vi "PatchExtractor.vi"(8 "error in":errorcluster caption="entrée d'erreur", 11 "PatchExtractor":T1={"patch_size"={"patch_height"=0, "patch_width"=0}, "max_patches"="None", "random_state"=-1} {"random_state" min=-1}) -> (0 "error out":errorcluster caption="sortie d'erreur", 3 "PatchExtractor.lvclass":refnum<class "PatchExtractor.lvclass">)   [LabVIEW 2020]
uses:
  PatchExtractor.lvclass
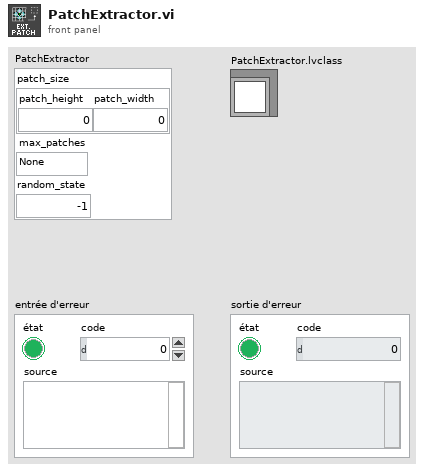
[diagram p1: front panel]
types:
  T1 = cluster{"patch_size":cluster{"patch_height":i32, "patch_width":i32}, "max_patches":string, "random_state":i32}
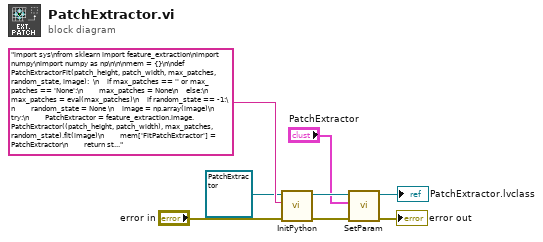
[diagram p0: block diagram]
diagram:
  n1 = call-dynamic "InitPython.vi"("error in (no error)"="error in", "Python Instruction"="import sys\nfrom sklearn import feature_extraction\nimport numpy\nimport numpy as np\n\n\nmem = {}\n\ndef PatchExtractorFit(patch_height, patch_width, max_patches, random_state, image):  \n    if max_patches == '' or max_patches == 'None':\n        max_patches = None\n    else:\n        max_patches = eval(max_patches)\n    if random_state == -1:\n        random_state = None \n    image = np.array(image)\n    try:\n        PatchExtractor = feature_extraction.image.PatchExtractor((patch_height, patch_width), max_patches, random_state).fit(image)\n        mem['FitPatchExtractor'] = PatchExtractor\n        return str('OK')\n    except:\n        erreur = sys.exc_info()\n        typerr = u\"%s\" % (erreur[0])\n        typerr = typerr[typerr.find(\"'\")+1:typerr.rfind(\"'\")]\n        msgerr = u\"%s\" % (erreur[1])\n        message = str('/!\\\\ {0} : {1}'. format(typerr,msgerr))\n        return message\n    \ndef PatchExtractorTransform(patch_height, patch_width, max_patches, random_state, image):  \n    if max_patches == '' or max_patches == 'None':\n        max_patches = None\n    else:\n        max_patches = eval(max_patches)\n    if random_state == -1:\n        random_state = None \n    image = np.array(image)\n    try:\n        Patches2D = mem['FitPatchExtractor'].transform(image)\n        Patches2Dlist = Patches2D.tolist()\n        return str(Patches2Dlist)\n    except:\n        erreur = sys.exc_info()\n        typerr = u\"%s\" % (erreur[0])\n        typerr = typerr[typerr.find(\"'\")+1:typerr.rfind(\"'\")]\n        msgerr = u\"%s\" % (erreur[1])\n        message = str('/!\\\\ {0} : {1}'. format(typerr,msgerr))\n        return message", "Scikit-learn en entrée"=refnum<class "PatchExtractor.lvclass"> refnum ("PatchExtractor.lvclass")) -> ("error out"=w5:errorcluster, "Scikit-learn en sortie"=w4:refnum<class "PatchExtractor.lvclass">)  [unwired: 7 in]
  n2 = call-dynamic "SetParam.vi"("error in (no error)"=w5, "PatchExtractor"="PatchExtractor", "PatchExtractor.lvclass"=w4) -> ("error out"=→"error out":errorcluster, "PatchExtractor.lvclass"=→"PatchExtractor.lvclass":refnum<class "PatchExtractor.lvclass">)  [unwired: 7 in]
